vi "init_hw.vi"(8 "error in (no error)":errorcluster, 11 "XPS control in":refnum<class "XPS.lvclass">) -> (0 "error out":errorcluster, 2 "Boolean":bool=TRUE, 3 "XPS control out":refnum<class "XPS.lvclass">)   [LabVIEW 2019, in "XPS.lvlib" / "XPS.lvclass"]
uses:
  XPS.lvclass
  XPS.lvclass/XPS.ctl
  Newport.XPS.CommandInterface
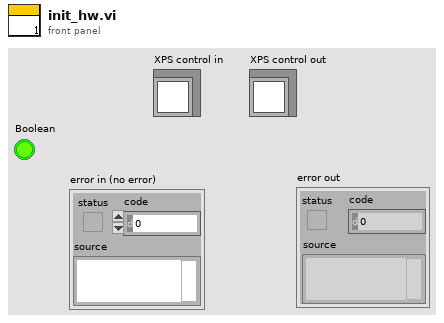
[diagram p1: front panel]
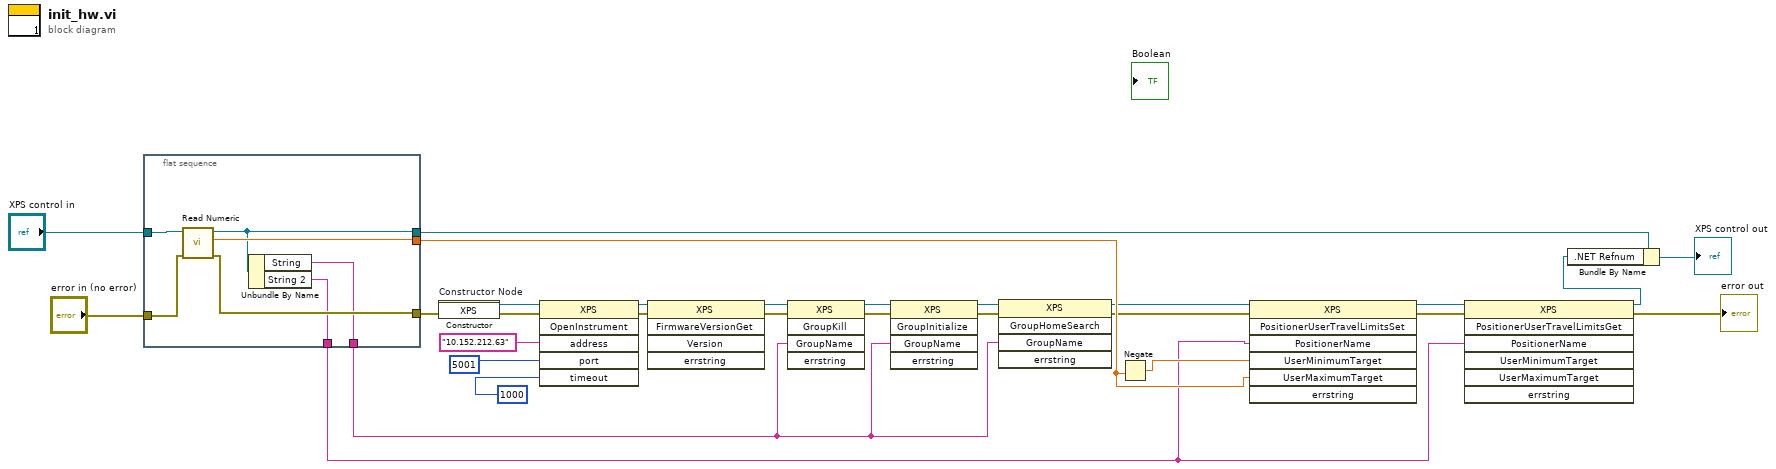
[diagram p0: block diagram]
diagram:
  n1 = flat-sequence {
    tunnel: [w31] -> _
    tunnel: [w35] -> w15
    tunnel: [w34] -> w9
    tunnel: "error in (no error)" -> [w33]
    tunnel: [w32] -> w6
    tunnel: "XPS control in" -> [w31]
    tunnel: [w30] -> w2
    tunnel: [w29] -> w1
    frame #0 {
      n2 = call-dynamic "Read Numeric.vi"("error in (no error)"=w33, "XPS in"=w31) -> ("error out"=w32:errorcluster, "Numeric"=w34:dbl, "XPS out"=w35:refnum<class "XPS.lvclass">)  [unwired: 7 in]
      n3 = Unbundle By Name(w31) -> ("String"=w30:string, "String 2"=w29:string)
    }
  }
  n4 = constructor on="Constructor Node" class="XPS"(error in=w6) -> (reference out=w23:refnum<k24>, error out=w27:errorcluster)  [unwired: 2 in, 1 out]
  n5 = invoke class="XPS" method="OpenInstrument"(reference=w23, error in=w27, "address"="10.152.212.63", "port"=5001, "timeout"=1000) -> (reference out=w26:refnum<k24>, error out=w28:errorcluster)  [unwired: 1 in, 4 out]
  n6 = invoke class="XPS" method="FirmwareVersionGet"(reference=w26, error in=w28) -> (reference out=w20:refnum<k24>, error out=w19:errorcluster)  [unwired: 3 in, 3 out]
  n7 = invoke class="XPS" method="GroupKill"(reference=w20, error in=w19, "GroupName"=w2) -> (reference out=w18:refnum<k24>, error out=w17:errorcluster)  [unwired: 2 in, 3 out]
  n8 = invoke class="XPS" method="GroupInitialize"(reference=w18, error in=w17, "GroupName"=w2) -> (reference out=w22:refnum<k24>, error out=w21:errorcluster)  [unwired: 2 in, 3 out]
  n9 = invoke class="XPS" method="GroupHomeSearch"(reference=w22, error in=w21, "GroupName"=w2) -> (reference out=w8:refnum<k24>, error out=w5:errorcluster)  [unwired: 2 in, 3 out]
  n10 = Negate(x=w9) -> (-x=w10:dbl)
  n11 = invoke class="XPS" method="PositionerUserTravelLimitsSet"(reference=w8, error in=w5, "PositionerName"=w1, "UserMinimumTarget"=w10, "UserMaximumTarget"=w9) -> (reference out=w14:refnum<k24>, error out=w13:errorcluster)  [unwired: 2 in, 5 out]
  n12 = invoke class="XPS" method="PositionerUserTravelLimitsGet"(reference=w14, error in=w13, "PositionerName"=w1) -> (reference out=w11:refnum<k24>, error out=→"error out":errorcluster)  [unwired: 4 in, 5 out]
  n13 = Bundle By Name(cluster=w15, ".NET Refnum"=w11) -> (→"XPS control out":refnum<class "XPS.lvclass">)
